vi "ReadCounters.vi"(0 "refnum":T1) -> (1 "refnum out":T1, 2 "Counters":T2(array[cluster]))   [LabVIEW 2018]
uses:
  <vilib>/Utility/config.llb/NI_LVConfig.lvlib
  <vilib>/Utility/config.llb/Read Key (String).vi
  <vilib>/Utility/config.llb/Config Data RefNum.ctl
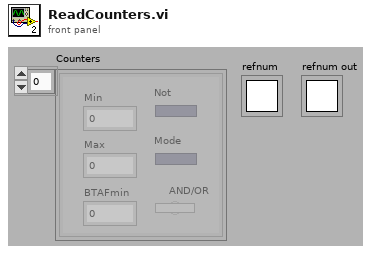
[diagram p1: front panel]
types:
  T1 = typedef "NI_LVConfig.lvlib/Config Data RefNum.ctl" = refnum<k1>
  T2 = cluster{"Min":i16, "Max":i16, "Not":bool, "Mode":bool, "BTAFmin":i16, "AND/OR":bool}[]
  T3 = cluster{"element":i16, "element":i16, bool, bool, "element":i16, bool}
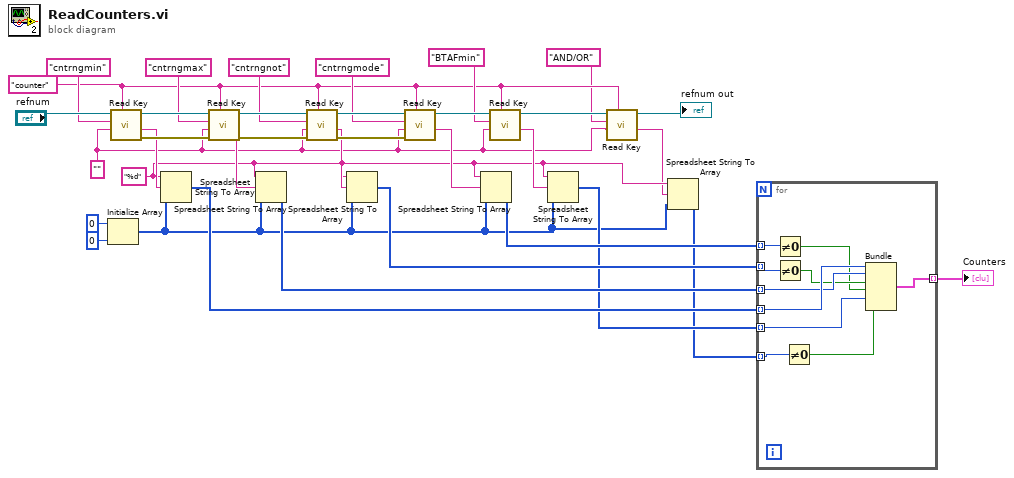
[diagram p0: block diagram]
diagram:
  w4 = "%d" ("format string")
  w6 = ""
  w8 = "counter" ("section")
  n1 = Initialize Array(i16 0 ("element"), 0 ("dimension size")) -> (w2:i16[])
  n2 = call-poly <vilib>:"Read Key.vi"("section"=w8, "default value"=w6, "key"="cntrngmin", "refnum"="refnum") -> ("error out"=w27:errorcluster, "value"=w24:string, "refnum out"=w33:T1)  [unwired: 4 in, 1 out]
  n3 = Spreadsheet String To Array(format string=w4, spreadsheet string=w24, array type (2D Dbl)=w2) -> (array=w14:i16[])  [unwired: 1 in]
  n4 = call-poly <vilib>:"Read Key.vi"("section"=w8, "error in (no error)"=w27, "default value"=w6, "key"="cntrngmax", "refnum"=w33) -> ("error out"=w26:errorcluster, "value"=w21:string, "refnum out"=w32:T1)  [unwired: 3 in, 1 out]
  n5 = Spreadsheet String To Array(format string=w4, spreadsheet string=w21, array type (2D Dbl)=w2) -> (array=w18:i16[])  [unwired: 1 in]
  n6 = call-poly <vilib>:"Read Key.vi"("section"=w8, "error in (no error)"=w26, "default value"=w6, "key"="cntrngnot", "refnum"=w32) -> ("error out"=w25:errorcluster, "value"=w20:string, "refnum out"=w31:T1)  [unwired: 3 in, 1 out]
  n7 = Spreadsheet String To Array(format string=w4, spreadsheet string=w20, array type (2D Dbl)=w2) -> (array=w17:i16[])  [unwired: 1 in]
  n8 = call-poly <vilib>:"Read Key.vi"("section"=w8, "error in (no error)"=w25, "default value"=w6, "key"="cntrngmode", "refnum"=w31) -> ("value"=w19:string, "refnum out"=w13:T1)  [unwired: 3 in, 2 out]
  n9 = Spreadsheet String To Array(format string=w4, spreadsheet string=w19, array type (2D Dbl)=w2) -> (array=w16:i16[])  [unwired: 1 in]
  n10 = call-poly <vilib>:"Read Key.vi"("section"=w8, "default value"=w6, "key"="BTAFmin", "refnum"=w13) -> ("value"=w11:string, "refnum out"=w9:T1)  [unwired: 4 in, 2 out]
  n11 = Spreadsheet String To Array(format string=w4, spreadsheet string=w11, array type (2D Dbl)=w2) -> (array=w10:i16[])  [unwired: 1 in]
  n12 = call-poly <vilib>:"Read Key.vi"("section"=w8, "default value"=w6, "key"="AND/OR", "refnum"=w9) -> ("value"=w3:string, "refnum out"=→"refnum out":T1)  [unwired: 4 in, 2 out]
  n13 = Spreadsheet String To Array(format string=w4, spreadsheet string=w3, array type (2D Dbl)=w2) -> (array=w1:i16[])  [unwired: 1 in]
  n14 = for {
    tunnel: w14 -> [w42] mode=indexing
    tunnel: w18 -> [w41] mode=indexing
    tunnel: w17 -> [w43] mode=indexing
    tunnel: w16 -> [w44] mode=indexing
    tunnel: [w45] -> w15 mode=indexing
    tunnel: w10 -> [w38] mode=indexing
    tunnel: w1 -> [w37] mode=indexing
    n15 = Not Equal To 0?(x=w44) -> (x != 0?=w39:bool)
    n16 = Not Equal To 0?(x=w43) -> (x != 0?=w40:bool)
    n17 = Not Equal To 0?(x=w37) -> (x != 0?=w36:bool)
    n18 = Bundle("element"=w42, "element"=w41, w40, w39, "element"=w38, w36) -> (w45:T3)  [unwired: 1 in]
  }
  "Counters" <- w15
